vi "query.vi"(8 "error in (no error)":errorcluster, 9 "Return Data (T)":bool=TRUE, 10 "Command Text":string, 11 "ADODB._Connection In":refnum<k7>) -> (0 "error out":errorcluster, 2 "Data":string[][](array[string]), 3 "ADODB._Connection Out":refnum<k7>)   [LabVIEW 2016, in "database.lvlib"]
uses:
  database.lvlib
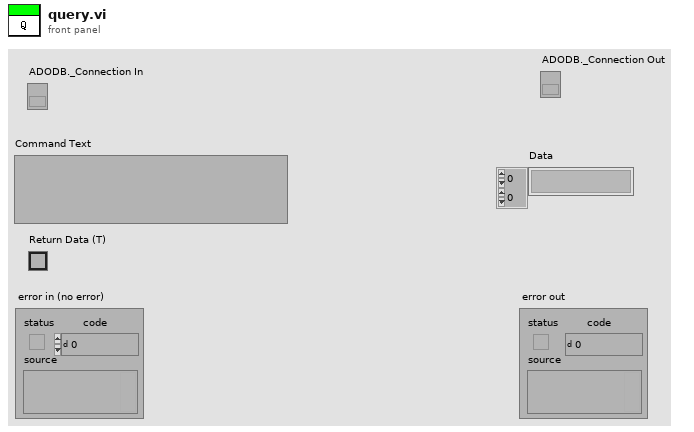
[diagram p1: front panel]
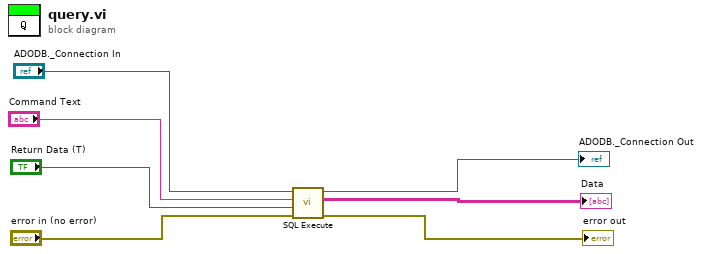
[diagram p0: block diagram]
diagram:
  n1 = call <userlib>:"SQL Execute.vi"("error in (no error)"="error in (no error)", "Return Data (T)"="Return Data (T)", "Command Text"="Command Text", "ADODB._Connection In"="ADODB._Connection In") -> ("error out"=→"error out":errorcluster, "Data"=→"Data":string[][], "ADODB._Connection Out"=→"ADODB._Connection Out":refnum<k7>)  [unwired: 4 in, 1 out]
